vi "Load_protocol.vi"(8 "error in (no error)":errorcluster, 11 "XML Elements":string) -> (0 "error IO":errorcluster, 3 "Protocol cluster":T1)   [LabVIEW 2016]
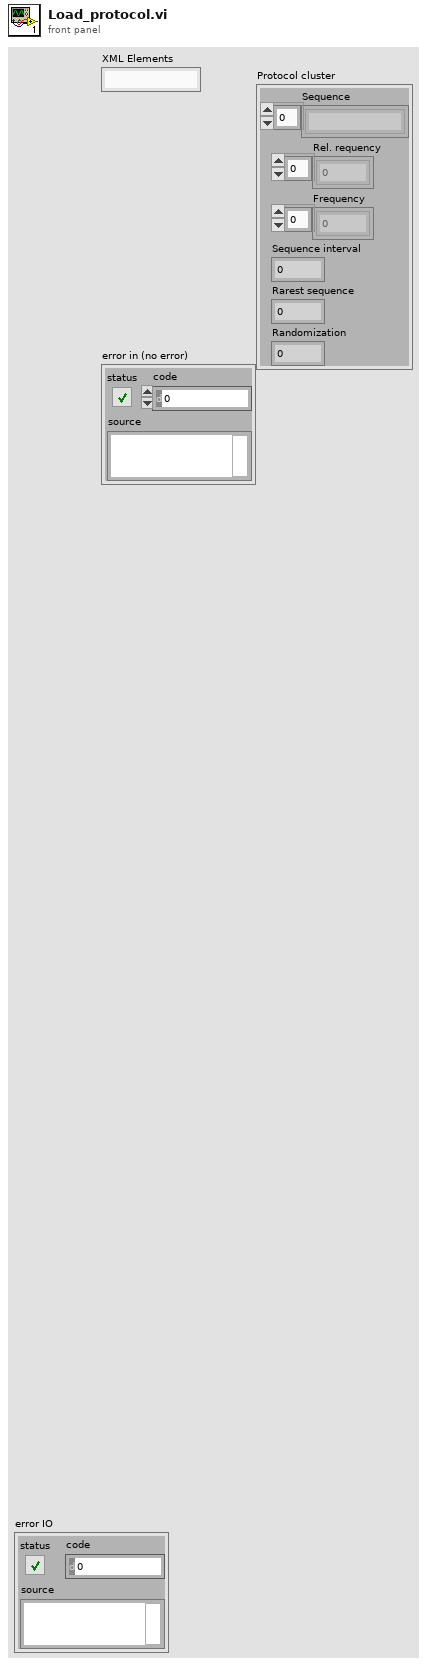
[diagram p1: front panel]
types:
  T1 = cluster{"Sequence":string[], "Rel. requency":dbl[], "Frequency":dbl[], "Sequence interval":dbl, "Rarest sequence ":dbl, "Randomization":u16}
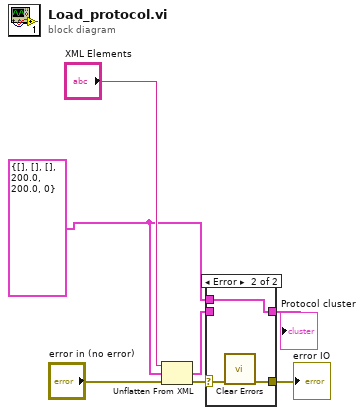
[diagram p0: block diagram]
diagram:
  w1 = T1 {"Sequence"=[], "Rel. requency"=[], "Frequency"=[], "Sequence interval"=200.0, "Rarest sequence "=200.0, "Randomization"=0} ("Protocol cluster")
  n1 = Unflatten From XML(xml string="XML Elements", type=w1, error in (no error)="error in (no error)") -> (value=w3:T1, error out=w5:errorcluster)
  n2 = case shown="Error" w5 {
    selector: w5 -> [w9 w12]
    tunnel: [w9 w11] -> w4
    tunnel: [w8 w10] -> w2
    tunnel: w3 -> [w8 _]
    tunnel: w1 -> [_ w10]
    frame No Error {
    }
    frame Error {
      n3 = call <vilib>:"Clear Errors.vi"("error in (no error)"=w12) -> ("error out"=w11:errorcluster)  [unwired: 5 in, 1 out]
    }
  }
  "error IO" <- w4
  "Protocol cluster" <- w2
